vi "Handle Messages.vi"(8 "error in (no error)":errorcluster, 9 "Message Data":variant, 10 "Message":string, 11 "Mock Async Handler Process In":refnum<class "Mock Async Handler Process.lvclass">) -> (0 "error out":errorcluster, 3 "Mock Async Handler Process Out":refnum<class "Mock Async Handler Process.lvclass">)   [LabVIEW 2020, in "Mock Async Handler Process.lvclass"]
uses:
  Mock Async Handler Process.lvclass
  C:/git/astemes-triarc-framework/source/Framework/Async Handler/Async Handler.lvclass
  source/Framework/Process/Process.lvclass
  Mock Async Handler Process.lvclass/Mock Async Handler Process.ctl
  source/Framework/Async Handler/Async Handler.lvclass
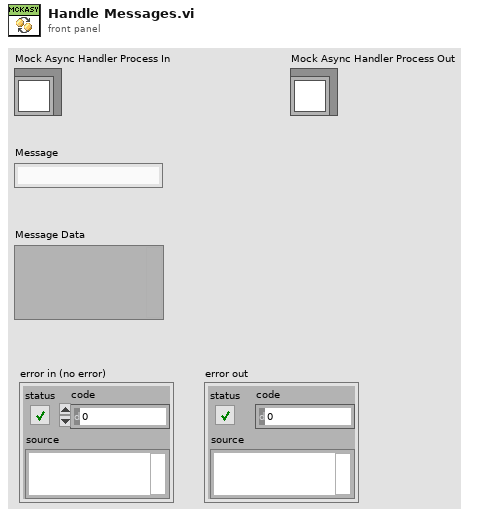
[diagram p1: front panel]
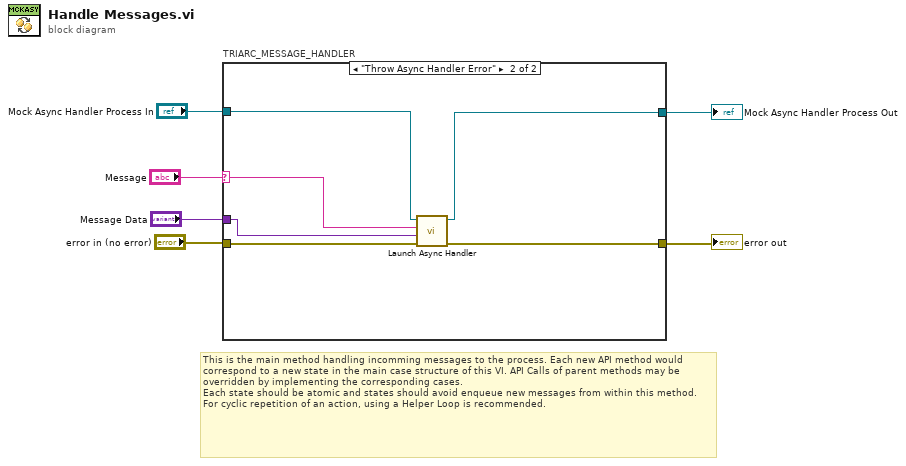
[diagram p0: block diagram]
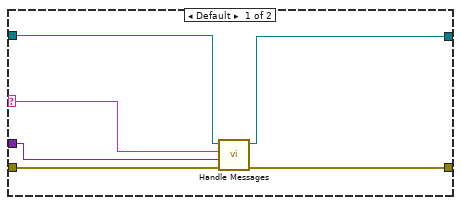
[diagram p2: hidden frame]
diagram:
  # "This is the main method handling incomming messages to the process. Each new API method would correspond to a new state in the main case structure of this VI. API Calls of parent methods may be overridden by implementing the corresponding cases.\nEach state should be atomic and states should avoid enqueue new messages from within this method. For cyclic repetition of an action, using a Helper Loop is recommended."
  n1 = case "TRIARC_MESSAGE_HANDLER" shown="\"Throw Async Handler Error\"" "Message" {
    selector: "Message" -> [w10 w16]
    tunnel: "error in (no error)" -> [w9 w14]
    tunnel: "Mock Async Handler Process In" -> [w12 w18]
    tunnel: "Message Data" -> [w11 w15]
    tunnel: [w8 w13] -> w2
    tunnel: [w7 w17] -> w1
    frame Default {
      n2 = call-parent "Handle Messages.vi"("error in (no error)"=w9, "Message Data"=w11, "Message"=w10, "Process In"=w12) -> ("error out"=w8:errorcluster, "Process Out"=w7:refnum<class "Mock Async Handler Process.lvclass">)  [unwired: 6 in]
    }
    frame "Throw Async Handler Error" {
      n3 = call "Launch Async Handler.vi"("error in (no error)"=w14, "Message Data"=w15, "Message"=w16, "Async Action In"=w18) -> ("error out"=w13:errorcluster, "Async Action Out"=w17:refnum<class "Mock Async Handler Process.lvclass">)  [unwired: 6 in]
    }
  }
  "error out" <- w2
  "Mock Async Handler Process Out" <- w1
